vi "Disable.vi"(8 "error in (no error)":errorcluster, 11 "Keysight44xx in":refnum<class "Keysight44xx.lvclass">) -> (0 "error out":errorcluster, 3 "Keysight44xx out":refnum<class "Keysight44xx.lvclass">)   [LabVIEW 2018, in "SpecAnPlugins.lvlib" / "Keysight44xx.lvclass"]
doc: "This VI places the instrument in a quiescent state where it has minimal or no impact on the system to which it is connected."
uses:
  Keysight44xx.lvclass
  C:/Users/ico/Documents/Projects/NistPluggableModules/SpecAn/SpecAnPlugins/SpecAnBaseClass/SpecAnBase.lvclass
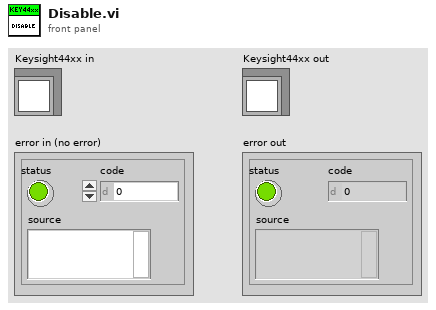
[diagram p1: front panel]
types:
  T1 = typedef "SpecAnPlugins.lvlib/SpecAnBase.lvclass/Acquisition.ctl" = cluster{"Handle":string, "Connected":bool, "Enabled":bool, "SweepModeContinuous":bool, "NumberOfSweeps":i32, "DetectorTypeAuto":bool, "DetectorType":i32, "VerticalScale":i32, "MaximumTime(seconds)":dbl}
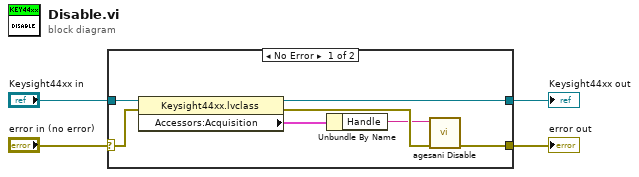
[diagram p0: block diagram]
diagram:
  n1 = case shown="No Error" "error in (no error)" {
    selector: "error in (no error)" -> [w10 w12]
    tunnel: "Keysight44xx in" -> [w11 w13]
    tunnel: [w9 w13] -> w2
    tunnel: [w5 w12] -> w1
    frame No Error {
      n2 = property class="Keysight44xx.lvclass"(reference=w11, error in=w10) -> (reference out=w9:refnum<class "Keysight44xx.lvclass">, error out=w7:errorcluster, "Accessors:Acquisition"=w8:T1)
      n3 = Unbundle By Name(w8) -> ("Handle"=w6:string)
      n4 = call <instrlib>:"agesani Disable.vi"("error in (no error)"=w7, "instrument handle"=w6) -> ("error out"=w5:errorcluster)  [unwired: 8 in, 1 out]
    }
    frame Error {
    }
  }
  "error out" <- w1
  "Keysight44xx out" <- w2
